vi "sub vi - Motor Step Imaging.vi"(7 "Left/Down":bool, 8 "Filename":string="C:\\Documents and Settings\\Peter\\Desktop\\test", 9 "# of Steps":dbl=10.0, 10 "Step Size":dbl=20.0, 11 "Axis":u16(ring) items=["X", "Y", "Z"]) -> (1 "Z  (7 in - 9 out)":dbl=-378.0, 2 "Y (-600-7000)":dbl=7095.0, 3 "X (-1000-1000)":dbl=-6372.0)   [LabVIEW 2010]
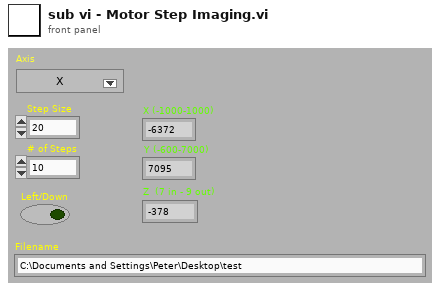
[diagram p1: front panel]
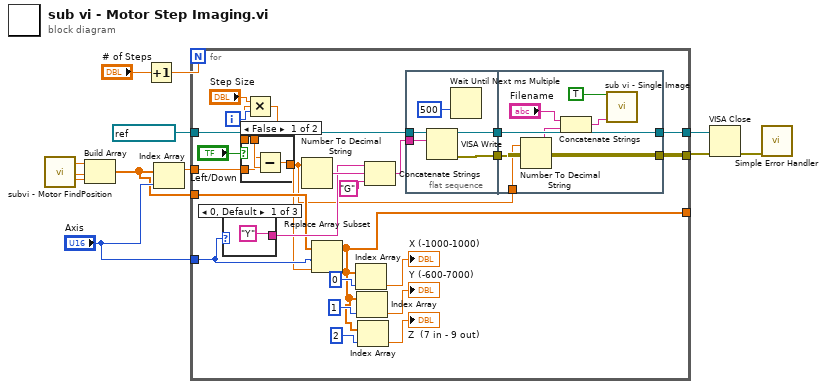
[diagram p0: block diagram]
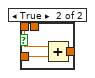
[diagram p2: hidden frame]
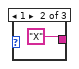
[diagram p3: hidden frame]
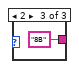
[diagram p4: hidden frame]
diagram:
  n1 = call "subvi - Motor FindPosition.vi"() -> ("X"=w5:dbl, "Y"=w4:dbl, "Z"=w3:dbl)  [unwired: 7 in, 10 out]
  n2 = Build Array(w5, w4, w3) -> (w2:dbl[])
  n3 = Increment(x="# of Steps") -> (x+1=w1:dbl)
  n4 = Index Array(array=w2, index="Axis") -> (element=w7:dbl)
  n5 = for {
    N: w1 -> [_]
    tunnel: refnum<visa-resource-name> "COM10" ("bottom (large beads)") -> [w36]
    tunnel: [w35] -> w10
    tunnel: [w34] -> w9
    tunnel: w7 -> [w19]
    tunnel: "Axis" -> [w24]
    tunnel: [w23] -> _
    tunnel: w2 -> [w18]
    i -> [w29]
    n6 = case shown="0, Default" w24 {
      tunnel: ["Y" "X" "8B"] -> w28
      frame 0, Default {
      }
      frame 1 {
      }
      frame 2 {
      }
    }
    n7 = Multiply(x="Step Size", y=w29) -> (x*y=w16:dbl)
    n8 = case shown="False" "Left/Down" {
      tunnel: w16 -> [_ w54]
      tunnel: [w51 w53] -> w13
      tunnel: w19 -> [w49 w52]
      tunnel: w16 -> [w50 _]
      frame False {
        n9 = Subtract(x=w49, y=w50) -> (x-y=w51:dbl)
      }
      frame True {
        n10 = Add(x=w54, y=w52) -> (x+y=w53:dbl)
      }
    }
    n11 = Number To Decimal String(number=w13) -> (decimal integer string=w32:string)  [unwired: 1 out]
    n12 = Replace Array Subset(array=w18, new element=w13, index=w24) -> (w23:dbl[])
    n13 = Index Array(array=w23, index=0) -> (element=→"X (-1000-1000)":dbl)
    n14 = Index Array(array=w23, index=1) -> (element=→"Y (-600-7000)":dbl)
    n15 = Index Array(array=w23, index=2) -> (element=→"Z  (7 in - 9 out)":dbl)
    n16 = Concatenate Strings(w28, w32, "G") -> (w31:string)
    n17 = flat-sequence {
      tunnel: w36 -> [w41]
      tunnel: w31 -> [w38]
      tunnel: [w40] -> w15
      tunnel: [w39] -> w14
      tunnel: [w47] -> w34
      tunnel: [w48] -> w35
      tunnel: w15 -> [w48]
      tunnel: w14 -> [w47]
      tunnel: w13 -> [w42]
      frame #0 {
        n18 = VISA Write(VISA resource name=w41, write buffer=w38) -> (VISA resource name out=w39:refnum<visa-resource-name>, error out=w40:errorcluster)  [unwired: 1 in, 1 out]
        n19 = Wait Until Next ms Multiple(millisecond multiple=u32 500) -> ()  [unwired: 1 out]
      }
      frame #1 {
        n20 = Number To Decimal String(number=w42) -> (decimal integer string=w43:string)  [unwired: 1 out]
        n21 = Concatenate Strings("Filename", w43) -> (w45:string)
        n22 = call "sub vi - Single Image.vi"("Filename"=w45, "save"=TRUE) -> ()  [unwired: 2 in, 8 out]
      }
    }
  }
  n23 = VISA Close(VISA resource name=w9, error in (no error)=w10) -> (error out=w11:errorcluster)
  n24 = call <vilib>:"Simple Error Handler.vi"("error in (no error)"=w11) -> ()  [unwired: 1 in, 8 out]
